vi "EMAPRE_NOTIF.vi"() -> ()   [LabVIEW 2015]
doc: "Uses the SMTP Email Client to send an email to a standard or secure SMTP server."
uses:
  <vilib>/smtpClient/SmtpClientHandle.ctl
  <vilib>/smtpClient/Set Message Text.vi
  <vilib>/smtpClient/LabVIEWSMTPClient.lvlib
panel:
  in  "Configure Server":bool
  in  "Sender's Email Address":string
  in  "Send Email":bool
  in  "Message":string
  in  "Subject":string
  in  "To:":string
  in  "Password":string
  in  "Enable TLS":bool
  in  "Username":string
  in  "Stop":bool
  in  "Port":string
  in  "Outgoing Mail Server (SMTP)":string
  # "Overview: Connects to an SMTP Email Server, and sends one or more emails.\nRequirements: LabVIEW Full Development System\nInstructions:\n1. Run the VI.\n2. Configure the Outgoing Mail Server section, then click Configure Server.\n3. Specify the Compose Email content, then click Send Email.\n4. Click Stop to stop the VI."
  # "Outgoing Mail Server"
  # "Compose Email"
  # "Optional Parameters"
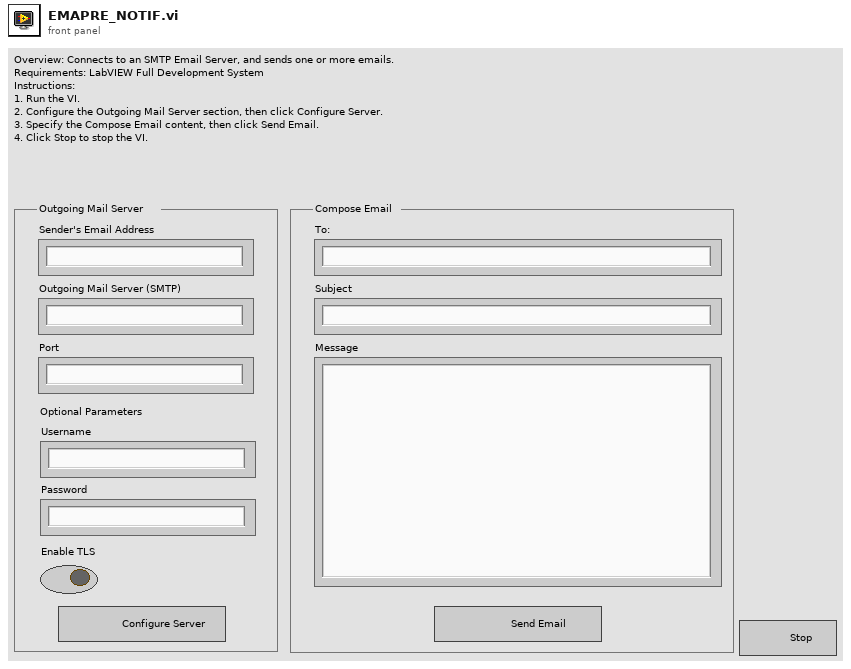
[diagram p1: front panel]
types:
  T1 = typedef "LabVIEWSMTPClient.lvlib/SmtpClientHandle.ctl" = refnum<k1>
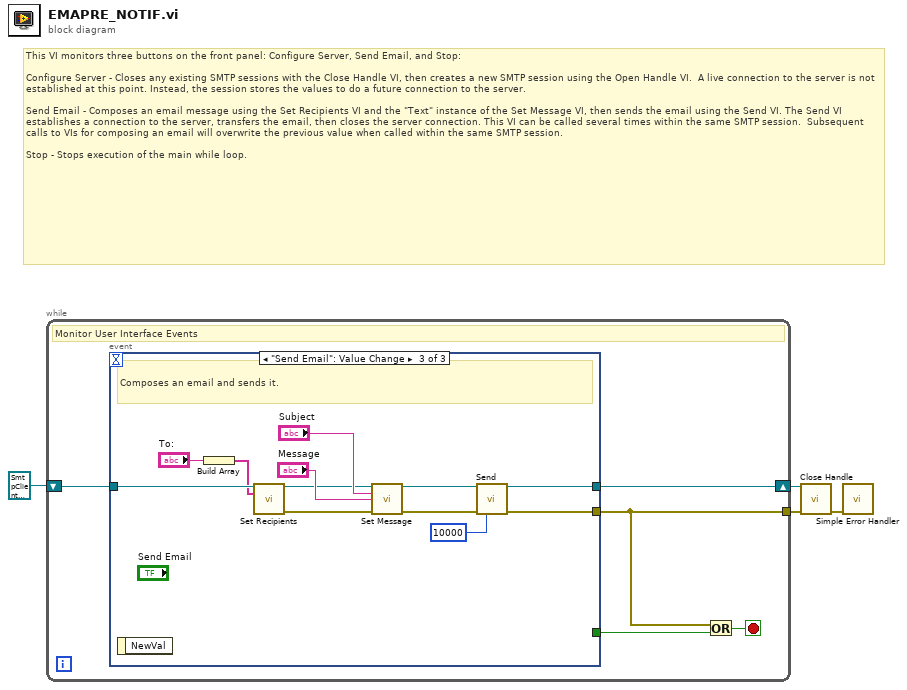
[diagram p0: block diagram]
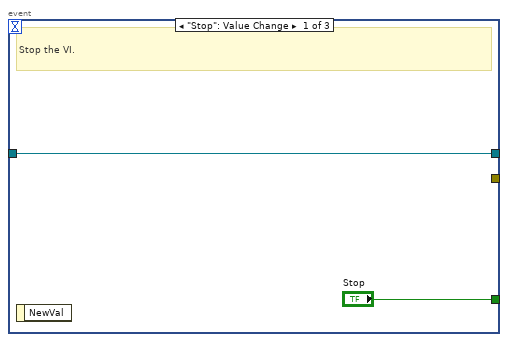
[diagram p2: hidden frame]
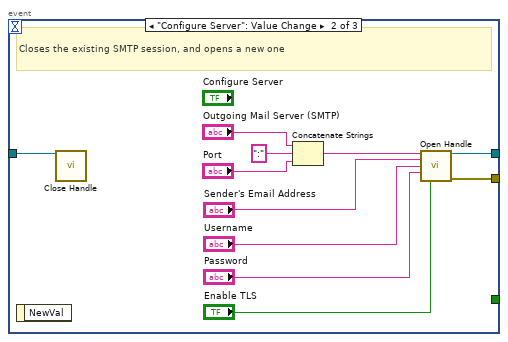
[diagram p3: hidden frame]
diagram:
  # "This VI monitors three buttons on the front panel: Configure Server, Send Email, and Stop:\n\nConfigure Server - Closes any existing SMTP sessions with the Close Handle VI, then creates a new SMTP session using the Open Handle VI.  A live connection to the server is not established at this point. Instead, the session stores the values to do a future connection to the server.\n\nSend Email - Composes an email message using the Set Recipients VI and the \"Text\" instance of the Set Message VI, then sends the email using the Send VI. The Send VI establishes a connection to the server, transfers the email, then closes the server connection. This VI can be called several times within the same SMTP session.  Subsequent calls to VIs for composing an email will overwrite the previous value when called within the same SMTP session.\n\nStop - Stops execution of the main while loop."
  n1 = while {
    shift-right: [w8] -> w4
    shift-left: T1 refnum ("handle out") -> [w9]
    tunnel: [w5] -> w2
    stop <- w7 stop-if-true
    # "Monitor User Interface Events"
    n2 = event shown="[2] \"Send Email\": Value Change" {
      selector: _ -> [_ _ _]
      dyn-events: _ -> [_ _ _]
      timeout: _ -> [_ _ _]
      tunnel: ["Stop" _ _] -> w6
      tunnel: w9 -> [w10 w13 w34]
      tunnel: [w10 w14 w25] -> w8
      tunnel: [_ w12 w23] -> w5
      event "Stop": Value Change {
        # "Stop the VI."
        n3 = event-data() -> ()  [unwired: 1 in, 1 out]
      }
      event "Configure Server": Value Change {
        # "Closes the existing SMTP session, and opens a new one"
        n4 = event-data() -> ()  [unwired: 1 in, 1 out]
        n5 = call <vilib>:"Close Handle.vi"("handle in"=w13) -> ()  [unwired: 13 in, 2 out]
        n6 = Concatenate Strings("Outgoing Mail Server (SMTP)", ":" ("string"), "Port") -> (w18:string)
        n7 = call <vilib>:"Open Handle.vi"("server address"=w18, "from"="Sender's Email Address", "username"="Username", "password"="Password", "use TLS (false)"="Enable TLS") -> ("handle out"=w14:T1, "error out"=w12:errorcluster)  [unwired: 9 in]
      }
      event "Send Email": Value Change {
        # "Composes an email and sends it."
        n8 = event-data() -> ()  [unwired: 1 in, 1 out]
        n9 = Build Array("To:") -> (w32:string[])
        n10 = call <vilib>:"Set Recipients.vi"("handle in"=w34, "to"=w32) -> ("handle out"=w28:T1, "error out"=w31:errorcluster)  [unwired: 12 in]
        n11 = call-poly <vilib>:"Set Message.vi"("handle in"=w28, "subject"="Subject", "plain text message"="Message", "error in (no error)"=w31) -> ("handle out"=w26:T1, "error out"=w27:errorcluster)  [unwired: 10 in]
        n12 = call <vilib>:"Send.vi"("handle in"=w26, "error in (no error)"=w27, "timeout in ms (10000)"=10000 ("timeout in ms")) -> ("handle out"=w25:T1, "error out"=w23:errorcluster)  [unwired: 10 in, 1 out]
      }
    }
    n13 = Or(x=w5, y=w6) -> (x .or. y?=w7:bool)
  }
  n14 = call <vilib>:"Close Handle.vi"("handle in"=w4, "error in (no error)"=w2) -> ("error out"=w1:errorcluster)  [unwired: 12 in, 1 out]
  n15 = call <vilib>:"Simple Error Handler.vi"("error in (no error)"=w1) -> ()  [unwired: 4 in, 5 out]
